vi "DecodeCANPayload.vi"(4 "ByteFormat":T1, 6 "DataFormat":T2, 11 "payload":u8[](array[numeric])) -> (3 "Value":sgl)   [LabVIEW 2016, in "DSI-RT.lvlib"]
uses:
  DSI-RT.lvlib
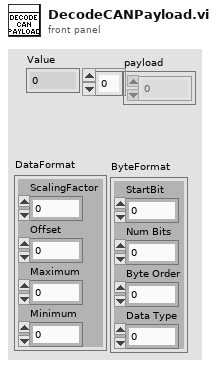
[diagram p1: front panel]
types:
  T1 = cluster{"StartBit":u8, "Num Bits":u8, "Byte Order":u8, "Data Type":u8}
  T2 = cluster{"ScalingFactor":sgl, "Offset":sgl, "Maximum":sgl, "Minimum":sgl}
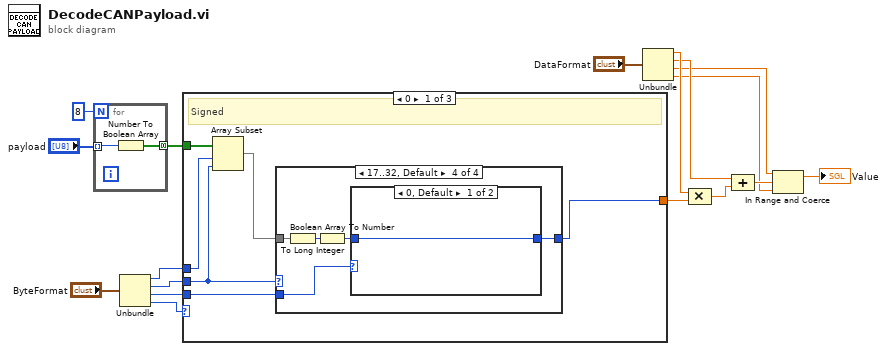
[diagram p0: block diagram]
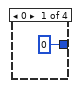
[diagram p2: hidden frame]
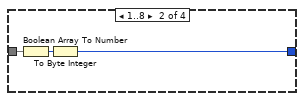
[diagram p3: hidden frame]
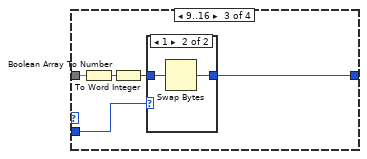
[diagram p4: hidden frame]
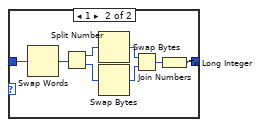
[diagram p6: hidden frame]
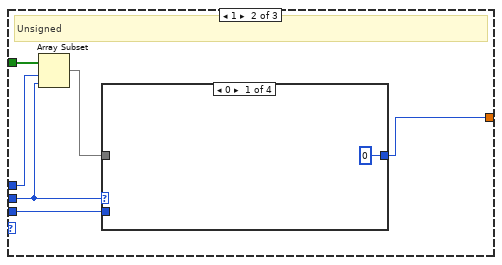
[diagram p7: hidden frame]
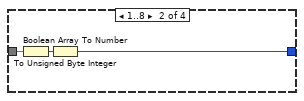
[diagram p8: hidden frame]
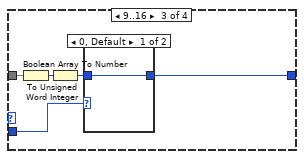
[diagram p9: hidden frame]
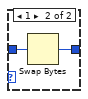
[diagram p10: hidden frame]
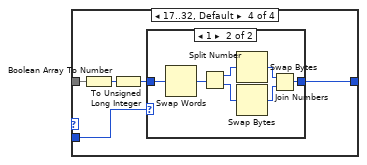
[diagram p11: hidden frame]
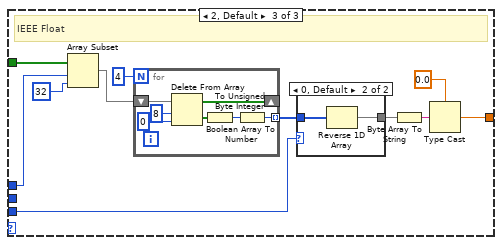
[diagram p13: hidden frame]
diagram:
  n1 = for {
    N: 8 -> [_]
    tunnel: "payload" -> [w19] mode=indexing
    tunnel: [w18] -> w9 mode=concatenating
    n2 = Number To Boolean Array(number=w19) -> (Boolean array=w18:bool[])
  }
  n3 = Unbundle("ByteFormat") -> ("StartBit"=w14:u8, "Num Bits"=w15:u8, "Byte Order"=w13:u8, "Data Type"=w11:u8)
  n4 = case shown="0" w11 {
    tunnel: w15 -> [w23 w55 _]
    tunnel: w14 -> [w22 w54 w92]
    tunnel: w9 -> [w24 w56 w93]
    tunnel: w13 -> [w25 w57 w91]
    tunnel: [w20 w52 w84] -> w8
    frame 0 {
      # "Signed"
      n5 = Array Subset(array=w24, index=w22, length=w23) -> (w21:bool[])
      n6 = case shown="17..32, Default" w23 {
        tunnel: w21 -> [_ w28 w32 w41]
        tunnel: [0 w27 w30 w38] -> w20
        tunnel: w25 -> [_ _ w34 w42]
        frame 0 {
        }
        frame 1..8 {
          n7 = Boolean Array To Number(Boolean array=w28) -> (number=w29:u32)
          n8 = To Byte Integer(number=w29) -> (8bit integer=w27:i8)
        }
        frame 9..16 {
          n9 = Boolean Array To Number(Boolean array=w32) -> (number=w31:u32)
          n10 = To Word Integer(number=w31) -> (16bit integer=w33:i16)
          n11 = case shown="1" w34 {
            tunnel: w33 -> [w35 w37]
            tunnel: [w35 w36] -> w30
            frame 0, Default {
            }
            frame 1 {
              n12 = Swap Bytes(anything=w37) -> (byte swapped=w36:i16)
            }
          }
        }
        frame 17..32, Default {
          n13 = Boolean Array To Number(Boolean array=w41) -> (number=w39:u32)
          n14 = To Long Integer(number=w39) -> (32bit integer=w40:i32)
          n15 = case shown="0, Default" w42 {
            tunnel: w40 -> [w43 w51]
            tunnel: [w43 w44] -> w38
            frame 0, Default {
            }
            frame 1 {
              n16 = Swap Words(1:w51) -> (0:w50:i32)
              n17 = Split Number(x=w50) -> (hi(x)=w49:u16, lo(x)=w48:u16)
              n18 = Swap Bytes(anything=w49) -> (byte swapped=w46:u16)
              n19 = Swap Bytes(anything=w48) -> (byte swapped=w47:u16)
              n20 = Join Numbers(hi=w46, lo=w47) -> ((hi.lo)=w45:u32)
              n21 = To Long Integer(number=w45) -> (32bit integer=w44:i32)
            }
          }
        }
      }
    }
    frame 1 {
      # "Unsigned"
      n22 = Array Subset(array=w56, index=w54, length=w55) -> (w53:bool[])
      n23 = case shown="0" w55 {
        tunnel: w53 -> [_ w60 w64 w73]
        tunnel: [u32 0 w59 w62 w70] -> w52
        tunnel: w57 -> [_ _ w66 w74]
        frame 0 {
        }
        frame 1..8 {
          n24 = Boolean Array To Number(Boolean array=w60) -> (number=w61:u32)
          n25 = To Unsigned Byte Integer(number=w61) -> (unsigned 8bit integer=w59:u8)
        }
        frame 9..16 {
          n26 = Boolean Array To Number(Boolean array=w64) -> (number=w63:u32)
          n27 = To Unsigned Word Integer(number=w63) -> (unsigned 16bit integer=w65:u16)
          n28 = case shown="0, Default" w66 {
            tunnel: w65 -> [w67 w69]
            tunnel: [w67 w68] -> w62
            frame 0, Default {
            }
            frame 1 {
              n29 = Swap Bytes(anything=w69) -> (byte swapped=w68:u16)
            }
          }
        }
        frame 17..32, Default {
          n30 = Boolean Array To Number(Boolean array=w73) -> (number=w71:u32)
          n31 = To Unsigned Long Integer(number=w71) -> (unsigned 32bit integer=w72:u32)
          n32 = case shown="1" w74 {
            tunnel: w72 -> [w75 w82]
            tunnel: [w75 w76] -> w70
            frame 0, Default {
            }
            frame 1 {
              n33 = Swap Words(1:w82) -> (0:w81:u32)
              n34 = Split Number(x=w81) -> (hi(x)=w80:u16, lo(x)=w79:u16)
              n35 = Swap Bytes(anything=w80) -> (byte swapped=w77:u16)
              n36 = Swap Bytes(anything=w79) -> (byte swapped=w78:u16)
              n37 = Join Numbers(hi=w77, lo=w78) -> ((hi.lo)=w76:u32)
            }
          }
        }
      }
    }
    frame 2, Default {
      # "IEEE Float"
      n38 = Array Subset(array=w93, index=w92, length=32) -> (w88:bool[])
      n39 = for {
        N: 4 -> [_]
        shift-right: [w99] -> _
        shift-left: w88 -> [w100]
        tunnel: [w95] -> w87 mode=indexing
        n40 = Delete From Array(array=w100, length=8, index=0) -> (deleted portion=w97:bool[], array with subset deleted=w99:bool[])
        n41 = Boolean Array To Number(Boolean array=w97) -> (number=w96:u32)
        n42 = To Unsigned Byte Integer(number=w96) -> (unsigned 8bit integer=w95:u8)
      }
      n43 = case shown="0, Default" w91 {
        tunnel: w87 -> [w101 w103]
        tunnel: [w101 w102] -> w86
        frame 1 {
        }
        frame 0, Default {
          n44 = Reverse 1D Array(array=w103) -> (reversed array=w102:u8[])
        }
      }
      n45 = Byte Array To String(unsigned byte array=w86) -> (string=w85:string)
      n46 = Type Cast(type=sgl 0.0, x=w85) -> (*(type *) &x=w84:sgl)
    }
  }
  n47 = Unbundle("DataFormat") -> ("ScalingFactor"=w7:sgl, "Offset"=w5:sgl, "Maximum"=w3:sgl, "Minimum"=w2:sgl)
  n48 = Compound Arithmetic op=MULTIPLY(w7, w8) -> (w6:sgl)
  n49 = Compound Arithmetic op=ADD(w5, w6) -> (w4:sgl)
  n50 = In Range and Coerce(upper limit=w3, x=w4, lower limit=w2) -> (coerced(x)=→"Value":sgl)  [unwired: 1 out]
